vi "angle_modulo.vi"(1 "alpha":dbl) -> (0 "alpha_prime":dbl)   [LabVIEW 2019]
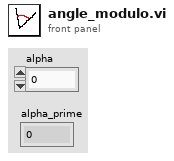
[diagram p1: front panel]
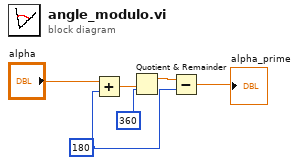
[diagram p0: block diagram]
diagram:
  w2 = 180
  n1 = Add(x="alpha", y=w2) -> (x+y=w5:dbl)
  n2 = Quotient & Remainder(x=w5, y=360) -> (x-y*floor(x/y)=w4:dbl)  [unwired: 1 out]
  n3 = Subtract(x=w4, y=w2) -> (x-y=→"alpha_prime":dbl)
